vi "Get LS DAS Data.vi"(8 "Initial LS Data":T1={"Total Cycles"=[0, 0, 0, 0, 0, 0], "Steps"=[0, 0, 0, 0, 0, 0], "Anomalies Total"=[0, 0, 0, 0, 0, 0], "Cycles"=[0, 0, 0, 0, 0, 0], "Anomalies/Cycle"=[0, 0, 0, 0, 0, 0], "Anomalies (Last Cycle)"=[0, 0, 0, 0, 0, 0], "Opens"=[0, 0, 0, 0, 0, 0]} {"Opens" format="%#.0f"; "Anomalies (Last Cycle)" format="%#.0f"; "Anomalies/Cycle" format="%#.0f"; "Cycles" format="%#.0f"; "Anomalies Total" format="%#.0f"; "Steps" format="%#.0f"; "Total Cycles" format="%#.0f"}, 11 "FPGA Ref":refnum<k20>) -> (3 "LS Data":T1 {"Opens" format="%#.0f"; "Anomalies (Last Cycle)" format="%#.0f"; "Anomalies/Cycle" format="%#.0f"; "Cycles" format="%#.0f"; "Anomalies Total" format="%#.0f"; "Steps" format="%#.0f"; "Total Cycles" format="%#.0f"})   [LabVIEW 2013]
uses:
  Type Defs/LS Data.ctl
  <vilib>/Utility/error.llb/Error Cluster From Error Code.vi
  <vilib>/rvi/errors/niLvFpgaAdjustHostInterfaceError.vi
  <vilib>/rvi/interface/nirviReadWriteControl/nirviReadWriteControl.xnode
  FPGA Bitfiles/LS Acquisition.lvbitx
  NiFpgaLv.dll
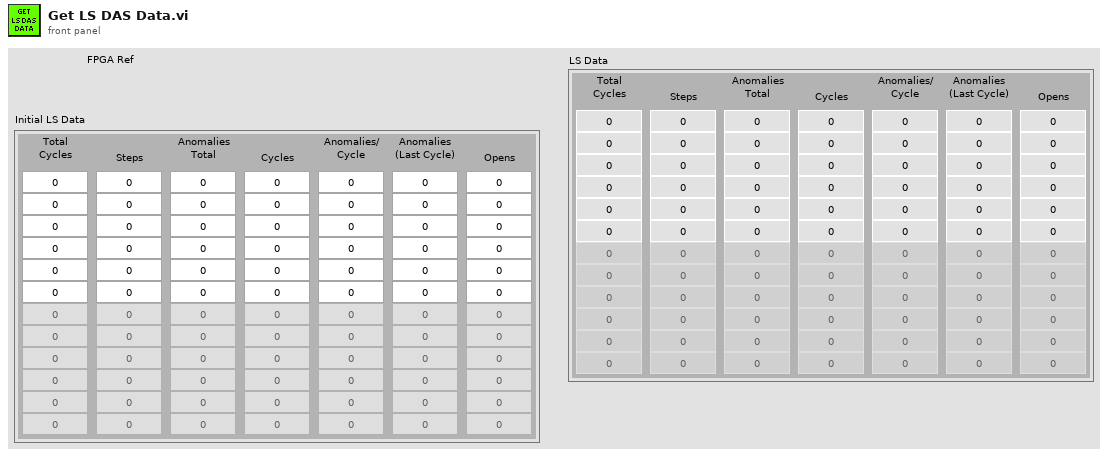
[diagram p1: front panel]
types:
  T1 = typedef "LS Data.ctl" = cluster{"Total Cycles":u32[], "Steps":u32[], "Anomalies Total":i32[], "Cycles":u32[], "Anomalies/Cycle":i32[], "Anomalies (Last Cycle)":i32[], "Opens":i32[]}
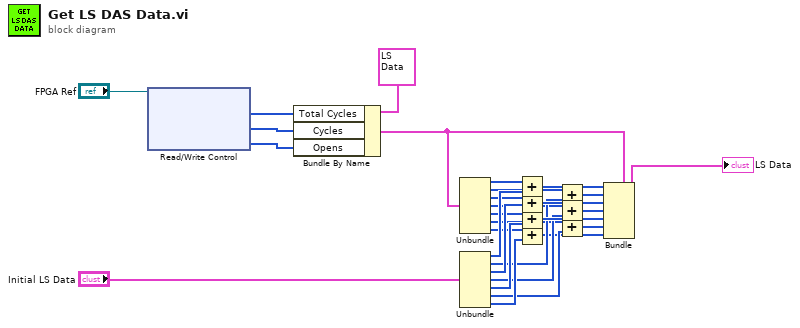
[diagram p0: block diagram]
diagram:
  n1 = xnode "Read/Write Control"("FPGA VI Reference In"="FPGA Ref") -> ("Total Cycles"=w28:u32[], "Cycles"=w3:u32[], "Opens Detected"=w2:u16[])  [unwired: 1 in, 2 out]
  n2 = Bundle By Name(cluster=T1 {"Total Cycles"=[0, 0, 0, 0, 0, 0, 0, 0, 0, 0, 0, 0], "Steps"=[0, 0, 0, 0, 0, 0, 0, 0, 0, 0, 0, 0], "Anomalies Total"=[0, 0, 0, 0, 0, 0, 0, 0, 0, 0, 0, 0], "Cycles"=[0, 0, 0, 0, 0, 0, 0, 0, 0, 0, 0, 0], "Anomalies/Cycle"=[0, 0, 0, 0, 0, 0, 0, 0, 0, 0, 0, 0], "Anomalies (Last Cycle)"=[0, 0, 0, 0, 0, 0, 0, 0, 0, 0, 0, 0], "Opens"=[]} ("LS Data"), "Total Cycles"=w28, "Cycles"=w3, "Opens"=w2) -> (w7:T1)
  n3 = Unbundle(w7) -> ("Total Cycles"=w8:u32[], "Steps"=w9:u32[], "Anomalies Total"=w10:i32[], "Cycles"=w11:u32[], "Anomalies/Cycle"=w12:i32[], "Anomalies (Last Cycle)"=w13:i32[], "Opens"=w14:i32[])
  n4 = Unbundle("Initial LS Data") -> ("Total Cycles"=w15:u32[], "Steps"=w16:u32[], "Anomalies Total"=w17:i32[], "Cycles"=w18:u32[], "Anomalies/Cycle"=w19:i32[], "Anomalies (Last Cycle)"=w20:i32[], "Opens"=w21:i32[])
  n5 = Add(x=w8, y=w15) -> (x+y=w22:u32[])
  n6 = Add(x=w10, y=w17) -> (x+y=w24:i32[])
  n7 = Add(x=w12, y=w19) -> (x+y=w26:i32[])
  n8 = Add(x=w14, y=w21) -> (x+y=w4:i32[])
  n9 = Add(x=w9, y=w16) -> (x+y=w23:u32[])
  n10 = Add(x=w11, y=w18) -> (x+y=w25:u32[])
  n11 = Add(x=w13, y=w20) -> (x+y=w27:i32[])
  n12 = Bundle(cluster=w7, "Total Cycles"=w22, "Steps"=w23, "Anomalies Total"=w24, "Cycles"=w25, "Anomalies/Cycle"=w26, "Anomalies (Last Cycle)"=w27, "Opens"=w4) -> (→"LS Data":T1)
